vi "AddTestMethod_CreateNewWizard_GetWeight.vi"(11 "Wizard":T1) -> (3 "Weight":i32)   [LabVIEW 2013]
uses:
  <resource>/Framework/Providers/API/ItemRef.ctl
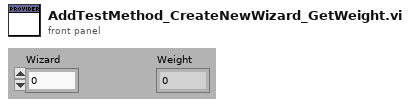
[diagram p1: front panel]
types:
  T1 = typedef "ItemRef.ctl" = u64
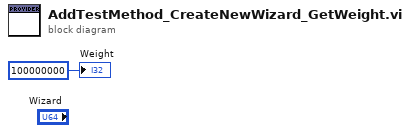
[diagram p0: block diagram]
diagram:
  "Weight" <- 100000000 ("Weight")
